vi "Surface Force Set.vi"(8 "error in (no error)":errorcluster, 9 "Force Constants":cluster{"k1":dbl, "k2":dbl, "k3":dbl, "k4":dbl}={"k1"=1.0, "k2"=1.0, "k3"=1.0, "k4"=1.0}, 10 "Force Settings":u16(ring) items=["0", "1", "2", "3", "4"]) -> (0 "error out":errorcluster)   [LabVIEW 2019, in "Haptic Prog Interface.lvlib"]
doc: "Returns the horizontal xy-position of the haptic pen in nm, and the vertical z-position in mm. The horizontal position depends on the frame origin and frame size.\n\n<b>Position:</b> Returns a cluster of the x (nm), y (nm), and z (mm) positions of the pen."
uses:
  Haptic Prog Interface.lvlib
  dll_path.vi
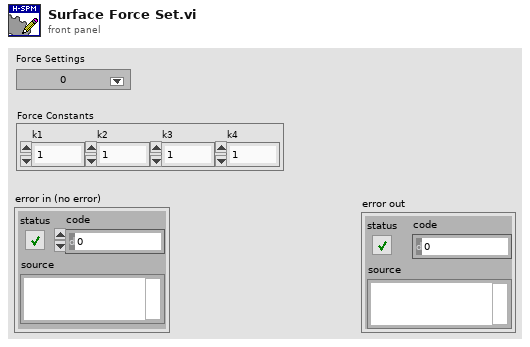
[diagram p1: front panel]
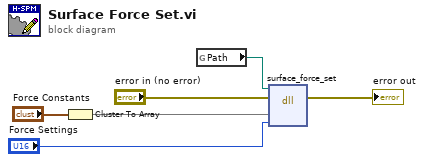
[diagram p0: block diagram]
diagram:
  n1 = Cluster To Array(cluster="Force Constants") -> (array=w2:dbl[])
  n2 = global read "dll_path.vi" "Path"() -> (w6:path)
  n3 = dll-call lib="C:/Users/freem/Documents/GitHub/HapticSPM/Haptic-Programming-Interface/x64/Release/Haptic Programming Interface.dll" fn="surface_force_set"(path in=w6, error in="error in (no error)", "input"=w2, "setting"="Force Settings") -> (error out=→"error out":errorcluster)  [unwired: 4 in, 1 out]
